vi "PYTHON Array Example.vi"() -> ()   [LabVIEW 2009]
uses:
  library/PYTHON Get String Data.vi
  library/PYTHON Get String Vector.vi
  library/PYTHON Get Float Matrix.vi
  library/PYTHON Set Float Matrix.vi
  library/PYTHON Set String Vector.vi
panel:
  out "strings out":string[](array[string])=["12", "23", "34", ""]
  out "string type":string="<type 'float'>"
  in  "strings":string[](array[string])=["12", "23", "34", ""]
  out "array out":dbl[][](array[numeric])=[[3.0], [4.0], [4.0], [5.0]] format="%.2f"
  in  "array":dbl[][](array[numeric])=[[11.0, 12.0, 13.0, 14.0], [21.0, 22.0, 23.0, 24.0]] format="%.2f"
  out "error out":errorcluster
  in  "error in (no error)":errorcluster
  in  "script":string="def listType1D(listToCheck=[]):\n    # check if empty list\n    if listToCheck == []:\n        return None\n    else:\n        #initialize sameTypes to TRUE\n        sameTypes = 1\n        #initialize listType to type of 1st element\n        listType = type(listToCheck[0])\n        #iterate thru list checking each elements type\n        for listElement in listToCheck:\n            # if same type then loop again\n            if type(listElement) == listType:\n                pass\n            #if not then break loop and return None\n            else:\n                sameTypes = 0\n                listType = None\n                break\n        # if loop completes then return the listType\n        return listType\n\nfloattype =  listType1D(floatmatrix)\nstringtype = listType1D(stringlist)"
  out "float type":string="<type 'float'>"
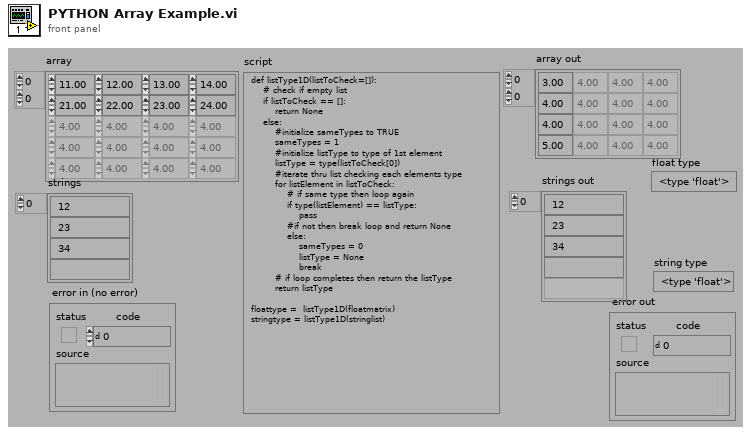
[diagram p1: front panel]
types:
  T1 = typedef "PYTHON Session Refnum.ctl" = refnum<k1>
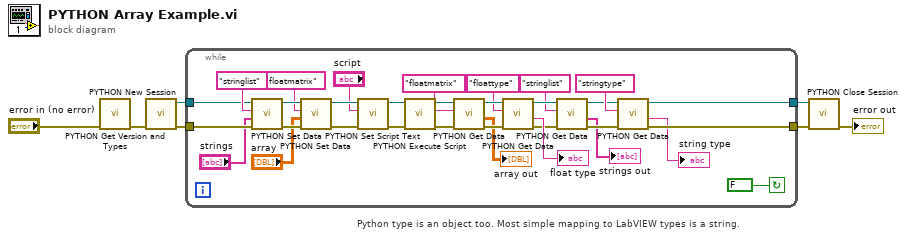
[diagram p0: block diagram]
diagram:
  # "Python type is an object too. Most simple mapping to LabVIEW types is a string."
  n1 = call "PYTHON Get Version and Types.vi"("error in (no error)"="error in (no error)") -> ("error out"=w5:errorcluster)  [unwired: 4 in, 2 out]
  n2 = call "PYTHON New Session.vi"("error in (no error)"=w5) -> ("error out"=w7:errorcluster, "Python Session"=w6:T1)  [unwired: 5 in]
  n3 = while {
    tunnel: w7 -> [w39]
    tunnel: w6 -> [w37]
    tunnel: [w12] -> w4
    tunnel: [w11] -> w3
    stop <- FALSE continue-if-true
    n4 = call-poly "PYTHON Set Data.vi"("error in (no error)"=w39, "value"="strings", "variable name"="stringlist", "Python Session in"=w37) -> ("error out"=w36:errorcluster, "Python Session out"=w35:T1)  [unwired: 2 in]
    n5 = call-poly "PYTHON Set Data.vi"("error in (no error)"=w36, "value"="array", "variable name"="floatmatrix", "Python Session in"=w35) -> ("error out"=w19:errorcluster, "Python Session out"=w33:T1)  [unwired: 2 in]
    n6 = call "PYTHON Set Script Text.vi"("error in (no error)"=w19, "script text"="script", "Python Session in"=w33) -> ("error out"=w30:errorcluster, "Python Session out"=w31:T1)  [unwired: 3 in]
    n7 = call "PYTHON Execute Script.vi"("error in (no error)"=w30, "Python Session in"=w31) -> ("error out"=w28:errorcluster, "Python Session out"=w29:T1)  [unwired: 4 in]
    n8 = call-poly "PYTHON Get Data.vi"("error in (no error)"=w28, "variable name"="floatmatrix", "Python Session in"=w29) -> ("error out"=w25:errorcluster, "value"=→"array out":dbl[][], "Python Session out"=w26:T1)  [unwired: 2 in]
    n9 = call-poly "PYTHON Get Data.vi"("error in (no error)"=w25, "variable name"="floattype", "Python Session in"=w26) -> ("error out"=w15:errorcluster, "value"=→"float type":string, "Python Session out"=w14:T1)  [unwired: 2 in]
    n10 = call-poly "PYTHON Get Data.vi"("error in (no error)"=w15, "variable name"="stringlist", "Python Session in"=w14) -> ("error out"=w13:errorcluster, "value"=→"strings out":string[], "Python Session out"=w16:T1)  [unwired: 2 in]
    n11 = call-poly "PYTHON Get Data.vi"("error in (no error)"=w13, "variable name"="stringtype", "Python Session in"=w16) -> ("error out"=w12:errorcluster, "value"=→"string type":string, "Python Session out"=w11:T1)  [unwired: 2 in]
  }
  n12 = call "PYTHON Close Session.vi"("error in (no error)"=w4, "Python Session in"=w3) -> ("error out"=→"error out":errorcluster)  [unwired: 5 in]
